vi "MoveThroughTo.vi"(6 "tolerances":dbl[][](array[numeric]), 8 "error in":errorcluster, 9 "speeds":dbl[](array[numeric]), 10 "accelerations":dbl[](array[numeric]), 11 "Poses":dbl[][][](array[numeric])) -> (0 "error out":errorcluster)   [LabVIEW 2013]
panel:
  in  "numPoses":i32
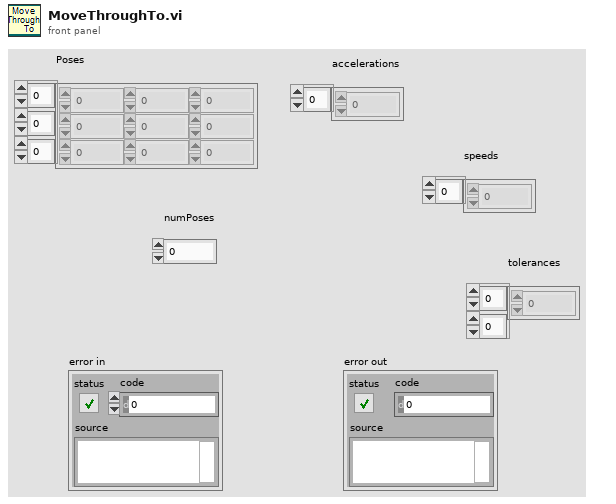
[diagram p1: front panel]
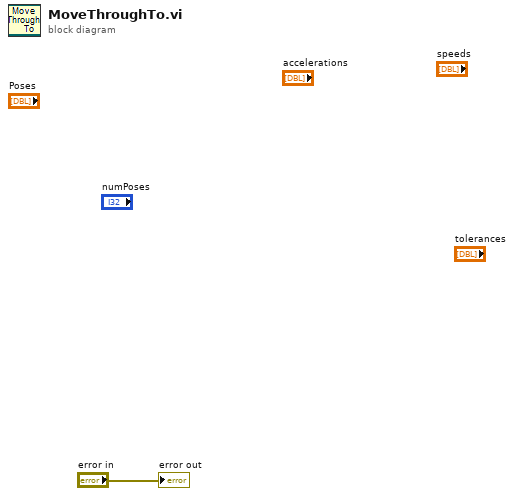
[diagram p0: block diagram]
diagram:
  "error out" <- "error in"
